vi "Gyro_Read.vi"(8 "error in":errorcluster, 9 "Gyro Sensitivity":T1=0.0175 items=["250 dps"=0.00875, "500 dps"=0.0175, "2000 dps"=0.07], 10 "Axis":T1 items=["X-Axis", "Y-Axis", "Z-Axis"], 11 "I2CDevRef":T2 {"Device Address" format="%.0x"}) -> (0 "error out":errorcluster, 1 "Heading":dbl, 2 "Rate":dbl, 3 "I2CDevRef Out":T2 {"Device Address" format="%.0x"})   [LabVIEW 2011]
uses:
  Gyro_Sensitivity.ctl
  <vilib>/Rock Robotics/WPI/I2C/WPI_I2CDevRef.ctl
  <vilib>/Rock Robotics/SystemInterfaces/Typedef/FPGA_TypedefDigitalModule.ctl
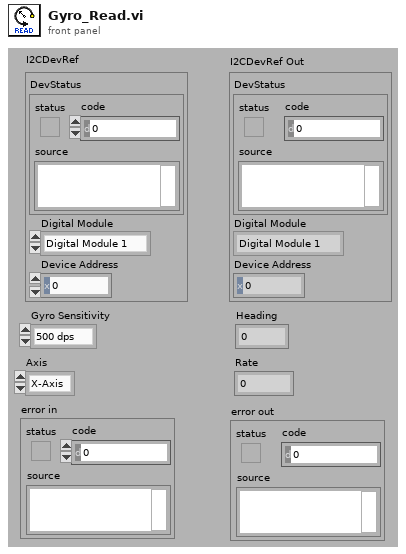
[diagram p1: front panel]
types:
  T1 = typedef "Gyro_Sensitivity.ctl" = dbl
  T2 = typedef "WPI_I2CDevRef.ctl" = cluster{"DevStatus":errorcluster, "Digital Module":T3, "Device Address":u8}
  T3 = typedef "FPGA_TypedefDigitalModule.ctl" = enum16{"Digital Module 1", "Digital Module 2"}
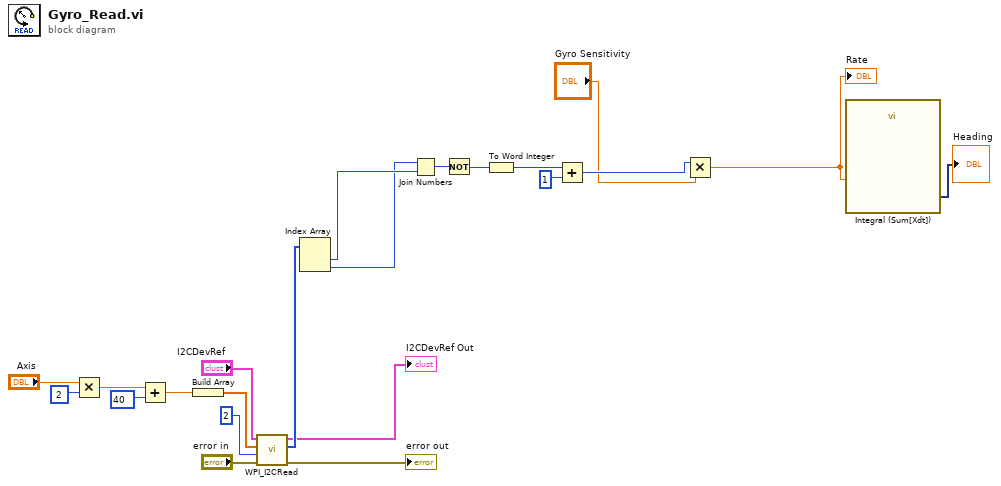
[diagram p0: block diagram]
diagram:
  n1 = Multiply(x="Axis", y=u8 2 ("Data To Send")) -> (x*y=w22:T1)
  n2 = Add(x=w22, y=u8 40 ("Data To Send")) -> (x+y=w11:T1)
  n3 = Build Array(w11) -> (w15:T1[])
  n4 = call <vilib>:"WPI_I2CRead.vi"("error in (no error)"="error in", "I2CBytesToRead"=u8 2, "I2CRegister"=w15, "I2CDevRef"="I2CDevRef") -> ("error out"=→"error out":errorcluster, "Data Out"=w14:u8[], "I2CDevRef"=→"I2CDevRef Out":T2)  [unwired: 1 in, 4 out]
  n5 = Index Array(array=w14) -> (element #1=w6:u8, element #2=w5:u8)  [unwired: 2 in]
  n6 = Join Numbers(hi=w5, lo=w6) -> ((hi.lo)=w3:u16)
  n7 = Not(x=w3) -> (.not. x?=w4:u16)
  n8 = To Word Integer(number=w4) -> (16bit integer=w18:i16)
  n9 = Add(x=w18, y=i16 1) -> (x+y=w2:i16)
  n10 = Multiply(x=w2, y="Gyro Sensitivity") -> (x*y=w7:T1)
  "Rate" <- w7
  n11 = call "Integral (Sum[Xdt])"("Signals"=w7) -> ("Result"=→"Heading":dynamicdata)  [unwired: 5 in, 1 out]
